vi "replaceUniquifierToken.vi"(8 "error in (no error)":errorcluster, 10 "Query In":string, 11 "Credit Transactions in":refnum<class "CreditTransactionList.lvclass">) -> (0 "error out":errorcluster, 2 "Query Out":string, 3 "Credit Transactions out":refnum<class "CreditTransactionList.lvclass">)   [LabVIEW 2018, in "CreditTransactionList.lvclass"]
uses:
  CreditTransactionList.lvclass
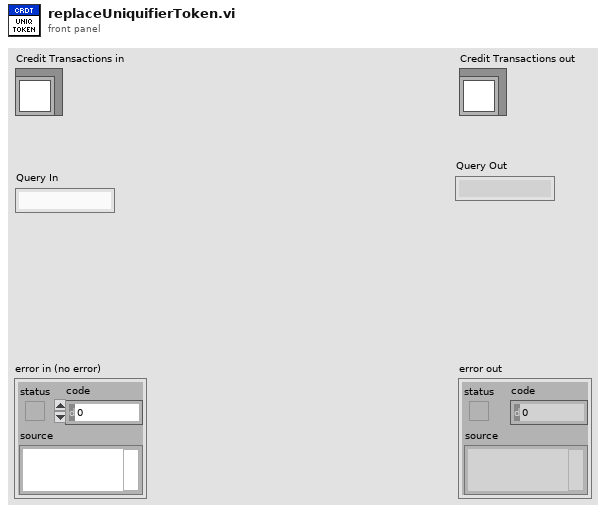
[diagram p1: front panel]
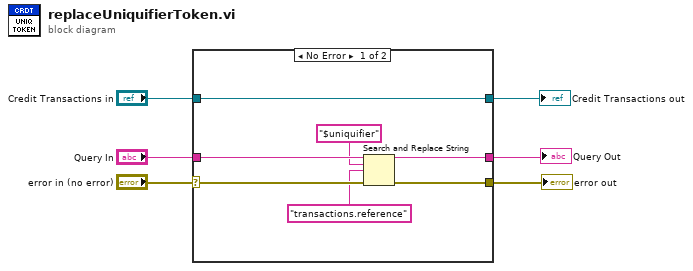
[diagram p0: block diagram]
diagram:
  n1 = case shown="No Error" "error in (no error)" {
    selector: "error in (no error)" -> [w11 w15]
    tunnel: [w10 w15] -> w1
    tunnel: [w13 w14] -> w2
    tunnel: "Credit Transactions in" -> [w13 w14]
    tunnel: "Query In" -> [w12 _]
    tunnel: [w9 _] -> w3
    frame No Error {
      n2 = Search and Replace String(input string=w12, search string="$uniquifier", replace string="transactions.reference", error in=w11) -> (result string=w9:string, error out=w10:errorcluster)  [unwired: 4 in, 2 out]
    }
    frame Error {
    }
  }
  "error out" <- w1
  "Credit Transactions out" <- w2
  "Query Out" <- w3
